vi "Get_measurnig_exp #.vi"(8 "error in (no error)":errorcluster, 11 "Control-Client in":refnum<class "Control-Client.lvclass">) -> (0 "error out":errorcluster, 2 "Exp measuring #":i32, 3 "Control-Client out":refnum<class "Control-Client.lvclass">)   [LabVIEW 2018, in "Control-Client.lvclass"]
uses:
  Control-Client.lvclass
  Control-Client.lvclass/Control-Client.ctl
  Experiments/Experiments_group.lvclass/Experiments_group.ctl
  methods/Read Group #.vi
  Experiments/Experiments_group.lvclass
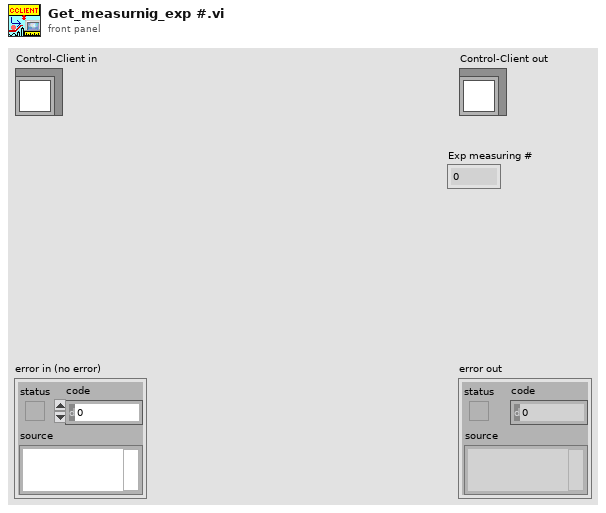
[diagram p1: front panel]
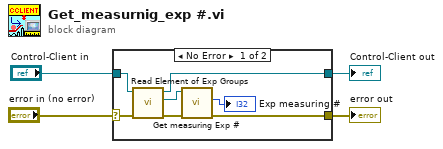
[diagram p0: block diagram]
diagram:
  n1 = case shown="No Error" "error in (no error)" {
    selector: "error in (no error)" -> [w10 w13]
    tunnel: [w7 w13] -> w3
    tunnel: [w9 w12] -> w1
    tunnel: "Control-Client in" -> [w11 w12]
    frame No Error {
      n2 = call "Read Element of Exp Groups.vi"("error in (no error)"=w10, "Control-Client in"=w11) -> ("error out"=w8:errorcluster, "Experiments_group.lvclass"=w6:refnum<class "Experiments_group.lvclass">, "Control-Client out"=w9:refnum<class "Control-Client.lvclass">)  [unwired: 7 in]
      n3 = call "Get measuring Exp #.vi"("error in (no error)"=w8, "Experiments_group in"=w6) -> ("error out"=w7:errorcluster, "Exp measuring #"=→"Exp measuring #":i32)  [unwired: 7 in, 1 out]
    }
    frame Error {
    }
  }
  "error out" <- w3
  "Control-Client out" <- w1
